vi "qSTA.vi"(0 "System no.":i32=1 min=1 max=4 step=1, 2 "Axes to query":string[](array[string]), 3 "All axes?":bool, 4 "Axis identifier?":bool=TRUE, 5 "error in":errorcluster) -> (14 "Axis status":dbl[](array[numeric]), 19 "error out":errorcluster)   [LabVIEW 2026]
doc: "Returns axis status (integer). Required by General wait for movement to stop.vi and Wait for axes to stop.vi.\n\nC702: If All axes = TRUE, then Axis identifier can be FALSE\nC-848: If All axes = TRUE, then Axis identifier can be FALSE\nC-880: If All axes = TRUE, then Axis identifier can be FALSE\nC-880K005: VI only supported when called through PI_Multix.vi\nC-886: Command is equivalent to #4. For details see user manual of the controller.\nC-887, F-206, M-8X0: All axes? = TRUE, Axis identifier? = FALSE. Command is equivalent to #4. For details see user manual of the controller."
panel:
  # "Returns axis status (integer)."
  # "If all axes: use"
  # "Query"
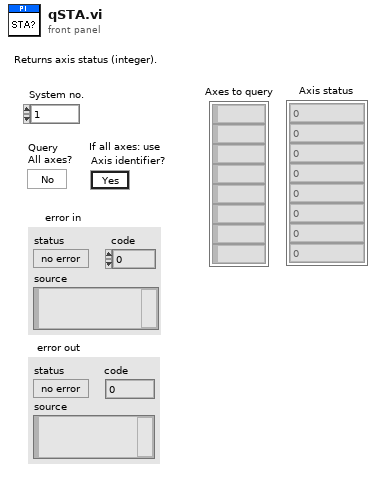
[diagram p1: front panel]
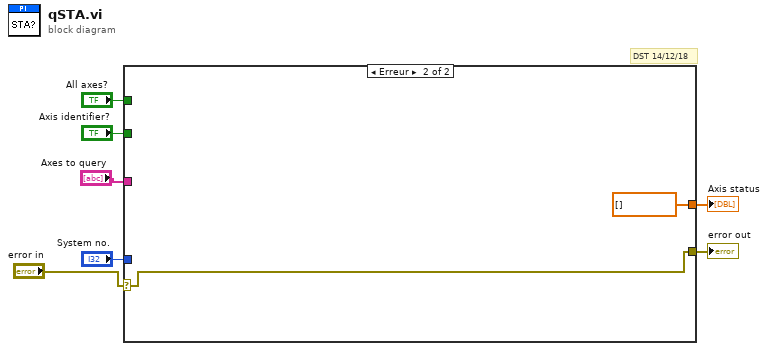
[diagram p0: block diagram]
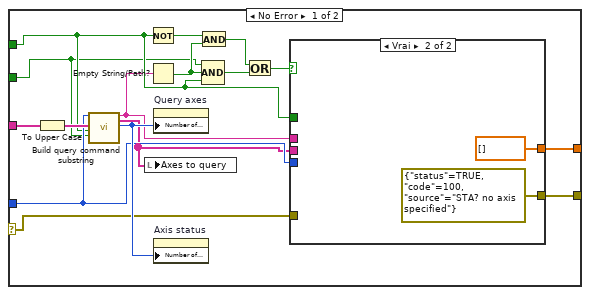
[diagram p2: hidden frame]
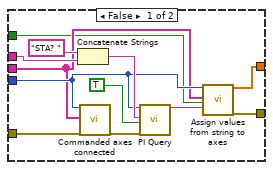
[diagram p3: hidden frame]
diagram:
  # "DST 14/12/18"
  n1 = case shown="Erreur" "error in" {
    selector: "error in" -> [w10 w38]
    tunnel: [w23 dbl[] [] ("Values")] -> w7
    tunnel: "Axes to query" -> [w22 _]
    tunnel: [w21 w38] -> w5
    tunnel: "System no." -> [w18 _]
    tunnel: "Axis identifier?" -> [w8 _]
    tunnel: "All axes?" -> [w14 _]
    frame No Error {
      n2 = To Upper Case(1:w22) -> (0:w20:string[])
      n3 = call "Build query command substring.vi"("System no."=w18, "Axes to query in"=w20, "Query\nAll axes?"=w14, "For all axes: use\nAxis identifier?"=w8) -> ("Command substring"=w11:string, "Axes to query out"=w17:string[], "Number of rows"=w19:u32)  [unwired: 2 in, 11 out]
      n4 = local write "Axes to query"(w17) -> ()
      n5 = Not(x=w14) -> (.not. x?=w16:bool)
      n6 = Empty String/Path?(string/path=w11) -> (empty?=w9:bool)
      n7 = property on="Query axes" class="Tabl (strict)"("Number of Rows"=w19) -> ()  [unwired: 2 in, 2 out]
      n8 = property on="Axis status" class="Tabl (strict)"("Number of Rows"=w19) -> ()  [unwired: 2 in, 2 out]
      n9 = And(x=w16, y=w9) -> (x .and. y?=w15:bool)
      n10 = Compound Arithmetic op=AND(w8, w9, w14) -> (w13:bool)
      n11 = Or(x=w15, y=w13) -> (x .or. y?=w12:bool)
      n12 = case shown="Vrai" w12 {
        tunnel: [w32 dbl[] [] ("Values")] -> w23
        tunnel: w10 -> [w31 _]
        tunnel: [w27 errorcluster {"status"=TRUE, "code"=100, "source"="STA? no axis specified"} ("error out")] -> w21
        tunnel: w11 -> [w30 _]
        tunnel: w18 -> [w29 _]
        tunnel: w17 -> [w28 _]
        tunnel: w14 -> [w26 _]
        frame False {
          n13 = Concatenate Strings("STA? ", w30) -> (w33:string)
          n14 = call "Commanded axes connected.vi"("System no."=w29, "Commanded axes"=w28, "error in"=w31) -> ("error out"=w25:errorcluster)  [unwired: 1 in, 15 out]
          n15 = call "PI Query.vi"("System no."=w29, "String to send"=w33, "Attach termination char.?"=TRUE ("Attach Linefeed?"), "error in"=w25) -> ("String read"=w24:string)  [unwired: 3 in, 12 out]
          n16 = call "Assign values from string to axes.vi"("System no."=w29, "Queried axes"=w28, "All axes queried?"=w26, "Input String"=w24) -> ("Values"=w32:dbl[], "error out"=w27:errorcluster)  [unwired: 5 in, 9 out]
        }
        frame True {
        }
      }
    }
    frame Error {
    }
  }
  "error out" <- w5
  "Axis status" <- w7
